vi "Arrange Tokens String.vi"(11 "Lib Tokens":string) -> (3 "Array":string[](array[string]))   [LabVIEW 2021, in "TAF Proj Document Type.lvlib" / "TAF Proj Config.lvclass"]
uses:
  <vilib>/Wovalab/AntiDoc/Document Type/Add-ons/LabVIEW TAF Project/TAF Proj Config/TAF Proj Config.lvclass
  <vilib>/Wovalab/AntiDoc/Document Type/Add-ons/LabVIEW TAF Project/TAF Proj Config/TAF Proj Config.lvclass/TAF Proj Config.ctl
  <vilib>/Wovalab/AntiDoc/Utilities/Utilities.lvlib
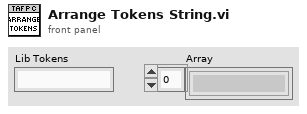
[diagram p1: front panel]
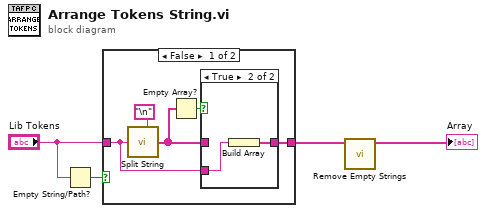
[diagram p0: block diagram]
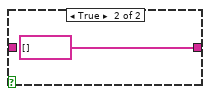
[diagram p3: hidden frame]
diagram:
  n1 = Empty String/Path?(string/path="Lib Tokens") -> (empty?=w3:bool)
  n2 = case shown="False" w3 {
    tunnel: [w7 string[] [] ("Split String")] -> w2
    tunnel: "Lib Tokens" -> [w5 _]
    frame False {
      n3 = call <vilib>:"Split String.vi"("Split Pattern"="\n", "Input String"=w5) -> ("Split String"=w6:string[])  [unwired: 5 in]
      n4 = Empty Array?(array=w6) -> (empty?=w8:bool)
      n5 = case shown="True" w8 {
        tunnel: [w10 w11] -> w7
        tunnel: w6 -> [w10 _]
        tunnel: w5 -> [_ w12]
        frame False {
        }
        frame True {
          n6 = Build Array(w12) -> (w11:string[])
        }
      }
    }
    frame True {
    }
  }
  n7 = call <vilib>:"Remove Empty Strings.vi"("Strings in"=w2) -> ("String out"=→"Array":string[])  [unwired: 10 in]
